vi "DAFDioTest.vi"() -> ()   [LabVIEW 2014]
uses:
  <vilib>/Platform/TimedLoop/XDataNode/wakeup.ctl
  <vilib>/Platform/TimedLoop/XDataNode/XDNodeRunTimeDep.lvlib
  <vilib>/Platform/TimedLoop/XDataNode/nitl_modes.ctl
  <vilib>/Platform/TimedLoop/XDataNode/timing_clust.ctl
  <vilib>/Platform/TimedLoop/XDataNode/XDataNode.xnode
  <vilib>/eio/EIONode/EIONode.xnode
  <vilib>/rvi/eio/common/nirviEmuTemplateMethod_errors.vi
panel:
  in  "Stop":bool
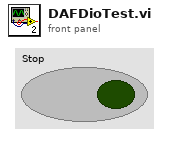
[diagram p1: front panel]
types:
  T1 = typedef "XDNodeRunTimeDep.lvlib/timing_clust.ctl" = cluster{"Expected End [f-1]":u64, "Actual End [f-1]":u64, "Finished Late? [f-1]":bool, "Expected End [i-1]":u64, "Actual End [i-1]":u64, "Finished Late? [i-1]":bool, "Expected Start [i]":u64, "Actual Start [i]":u64, "Expected Start [f]":u64, "Actual Start [f]":u64, "Source Name":string, "Structure Name":string, "Period":i64, "Deadline":i64, "Offset":i64, "Start":i64, "Priority":i32, "Timeout":i32, "Mode":T2, "Wakeup Reason":T3, "Error":errorcluster, "Source Type":string, "Secondary Source Type":string, "Global End Time":u64, "Global Start Time":u64, "Frame Duration":u64, "Iteration Duration":u64, "Assigned CPU":i32, "I/O Scan Engine Mode":u32}
  T2 = typedef "XDNodeRunTimeDep.lvlib/nitl_modes.ctl" = enum32{"No Change", "Process missed periods, maintain original phase", "Discard missed periods, maintain original phase", "Process missed periods, ignore original phase", "Discard missed periods, ignore original phase"}
  T3 = typedef "XDNodeRunTimeDep.lvlib/wakeup.ctl" = enum32{"Normal", "Aborted", "Asynchronous wakeup", "Timing source error", "Timed loop error", "Timeout"}
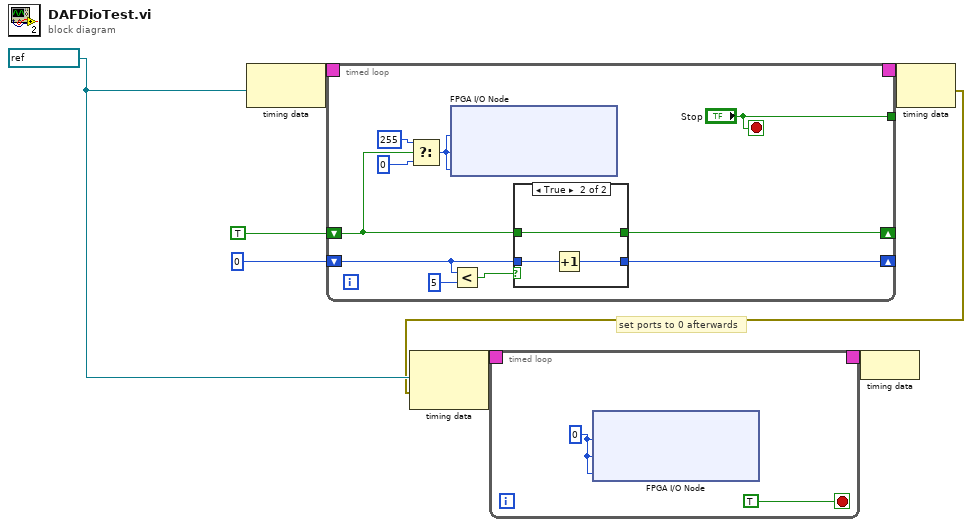
[diagram p0: block diagram]
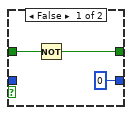
[diagram p2: hidden frame]
diagram:
  w4 = refnum<k21> "100MHz" ("Source Name")
  # "set ports to 0 afterwards"
  n1 = node-c288(w4) -> (w8:T1)
  n2 = timed-loop {
    timing: w8 -> [_]
    timing-out: [_] -> w7
    tunnel: ["Stop"] -> _
    shift-right: [w9] -> _
    shift-left: TRUE -> [w10]
    shift-right: [w14] -> _
    shift-left: u8 0 -> [w13]
    stop <- "Stop" stop-if-true
    n3 = Select(t=u8 255, s=w10, f=u8 0) -> (s? t:f=w17:u8)
    n4 = xnode "FPGA I/O Node"("Connector1/DIOPORT0"=w17, "Connector1/DIOPORT1"=w17, "Connector1/DIOPORT2"=w17) -> ()  [unwired: 3 in, 3 out]
    n5 = Less?(x=w13, y=u8 5) -> (x < y?=w12:bool)
    n6 = case shown="True" w12 {
      tunnel: w13 -> [_ w24]
      tunnel: [u8 0 w23] -> w14
      tunnel: w10 -> [w20 w22]
      tunnel: [w19 w22] -> w9
      frame False {
        n7 = Not(x=w20) -> (.not. x?=w19:bool)
      }
      frame True {
        n8 = Increment(x=w24) -> (x+1=w23:u8)
      }
    }
  }
  n9 = node-c288(w7) -> (w3:errorcluster)
  n10 = node-c288(w4, w3) -> (w6:T1)
  n11 = timed-loop {
    timing: w6 -> [_]
    timing-out: [_] -> w5
    stop <- TRUE stop-if-true
    w28 = u8 0
    n12 = xnode "FPGA I/O Node"("Connector1/DIOPORT0"=w28, "Connector1/DIOPORT1"=w28, "Connector1/DIOPORT2"=w28) -> ()  [unwired: 3 in, 3 out]
  }
  n13 = node-c288(w5) -> ()
